vi "DSF.Engine.Builder.Create.vi"(8 "error in (no error)":errorcluster, 10 "Framework Cache":refnum<class "DSF.Engine.Memory.Cache.Framework.lvclass">, 11 "Builder type":refnum<class "DSF.Engine.Builder.lvclass">) -> (0 "error out":errorcluster, 3 "Builder":refnum<class "DSF.Engine.Builder.lvclass">)   [LabVIEW 2016, in "DSF.Engine.lvlib" / "DSF.Engine.Builder.lvclass"]
uses:
  DSF.Engine.Builder.lvclass
  Cache/DSF.Engine.Memory.Cache.Framework.lvclass
  DSF.Engine.Builder.lvclass/DSF.Engine.Builder.ctl
  Interface/DSF.Engine.Interface.Builder.lvclass
  Status/Status.Builder.lvclass
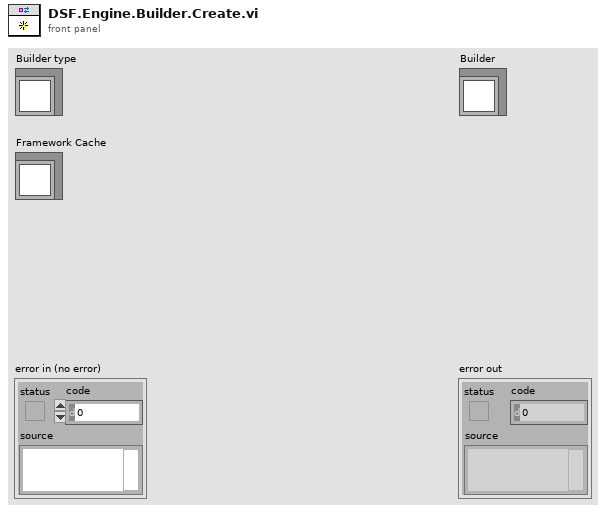
[diagram p1: front panel]
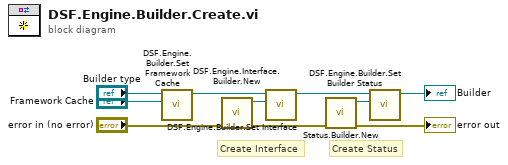
[diagram p0: block diagram]
diagram:
  # "Create Status"
  # "Create Interface"
  n1 = call "DSF.Engine.Builder.Set Framework Cache.vi"("Framework Cache"="Framework Cache", "Builder in"="Builder type") -> ("Builder out"=w1:refnum<class "DSF.Engine.Builder.lvclass">)  [unwired: 9 in]
  n2 = call "DSF.Engine.Interface.Builder.New.vi"("error in (no error)"="error in (no error)") -> ("error out"=w4:errorcluster, "Builder Interface"=w8:refnum<class "DSF.Engine.Interface.Builder.lvclass">)  [unwired: 9 in]
  n3 = call "DSF.Engine.Builder.Set Interface.vi"("Builder Interface"=w8, "Builder in"=w1) -> ("Builder out"=w6:refnum<class "DSF.Engine.Builder.lvclass">)  [unwired: 9 in]
  n4 = call "Status.Builder.New.vi"("error in (no error)"=w4) -> ("error out"=→"error out":errorcluster, "Builder Status"=w5:refnum<class "Status.Builder.lvclass">)  [unwired: 9 in]
  n5 = call "DSF.Engine.Builder.Set Builder Status.vi"("Builder Status"=w5, "Builder in"=w6) -> ("Builder out"=→"Builder":refnum<class "DSF.Engine.Builder.lvclass">)  [unwired: 9 in]
